vi "Events.vi"(11 "GUI Element in":refnum<class "GUI Element.lvclass">) -> (2 "Events":T1[](array[typedef]))   [LabVIEW 2020, in "VolatusGUI.lvlib" / "GUI Element.lvclass"]
uses:
  GUI Element.lvclass
  GUI Element.lvclass/GUI Element.ctl
  Control Event Registrations/Control Event Registrations.lvclass
  Control Event.ctl
  VolatusGUI.lvlib
  Event Registration.ctl
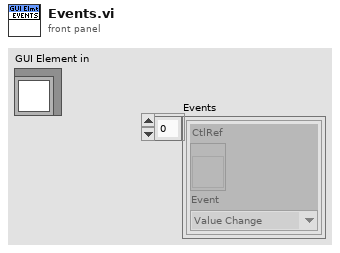
[diagram p1: front panel]
types:
  T1 = typedef "VolatusGUI.lvlib/Event Registration.ctl" = cluster{"CtlRef":refnum<vi>, "Event":T2}
  T2 = typedef "VolatusGUI.lvlib/Control Event.ctl" = enum16{"Value Change", "Shortcut Menu", "Mouse Down"}
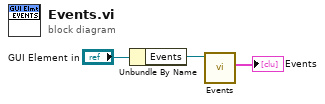
[diagram p0: block diagram]
diagram:
  n1 = Unbundle By Name("GUI Element in") -> ("Events"=w3:refnum<class "Control Event Registrations.lvclass">)
  n2 = call "Events.vi"("Control Event Registrations in"=w3) -> ("Events"=→"Events":T1[])  [unwired: 10 in]
